vi "파일경로(샘플00).vi"() -> ()   [LabVIEW 2014]
panel:
  out "에러 출력":errorcluster
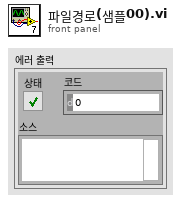
[diagram p1: front panel]
types:
  T1 = enum16{"open", "replace", "create", "open or create", "replace or create", "replace or create with confirmation"}
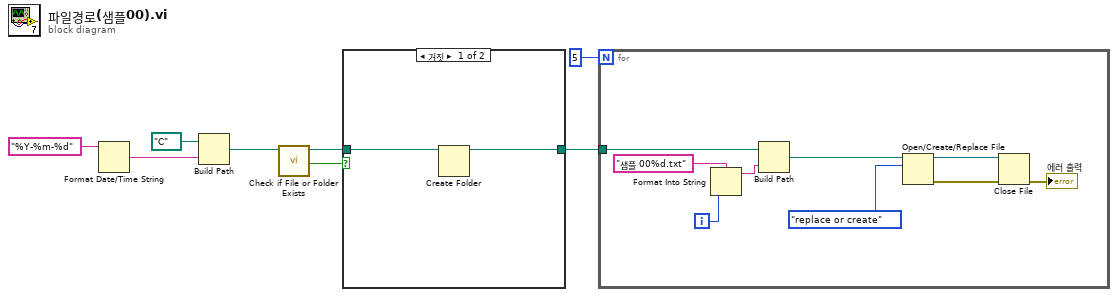
[diagram p0: block diagram]
diagram:
  n1 = Format Date/Time String(time format string (%c)="%Y-%m-%d" ("시간 포맷 문자열 (%c)")) -> (date/time string=w7:string)  [unwired: 2 in]
  n2 = Build Path(base path=path "C:/" ("베이스 경로"), name or relative path=w7) -> (appended path=w6:path)
  n3 = call <vilib>:"Check if File or Folder Exists.vi"("path"=w6) -> ("file or folder exists?"=w3:bool, "dup path"=w5:path)  [unwired: 8 in, 1 out]
  n4 = case shown="거짓" w3 {
    tunnel: w5 -> [w10 w11]
    tunnel: [w9 w11] -> w4
    frame False {
      n5 = Create Folder(path (use dialog)=w10) -> (created path=w9:path)  [unwired: 2 in, 2 out]
    }
    frame True {
    }
  }
  n6 = for {
    N: 5 -> [_]
    tunnel: w4 -> [w20]
    i -> [w14]
    n7 = Format Into String(format string="샘플 00%d.txt" ("초기 문자열"), w14) -> (resulting string=w13:string)  [unwired: 2 in, 1 out]
    n8 = Build Path(base path=w20, name or relative path=w13) -> (appended path=w19:path)
    n9 = Open/Create/Replace File(file path (use dialog)=w19, operation (0:open)=T1."replace or create" ("동작(0:open)")) -> (refnum out=w17:refnum<file>, error out=w16:errorcluster)  [unwired: 4 in, 1 out]
    n10 = Close File(refnum=w17, error in=w16) -> (error out=→"에러 출력":errorcluster)  [unwired: 1 out]
  }
